vi "calcUkRef0.vi"(8 "error in (no error)":errorcluster, 9 "dofIdx":i32[](array[numeric]), 10 "Qx Array":dbl[][](array[numeric]), 11 "OptCtrl in":refnum<class "OptCtrl.lvclass">) -> (0 "error out":errorcluster, 2 "uk Array":dbl[](array[numeric]), 3 "OptCtrl out":refnum<class "OptCtrl.lvclass">)   [LabVIEW 2016, in "OptCtrl.lvclass"]
doc: "Calculate uk by referencing to \"0\". The offset will trace the real value and target for 0."
uses:
  OptCtrl.lvclass
  OptCtrl.lvclass/OptCtrl.ctl
  <vilib>/Analysis/baseanly.llb/Real A x B.vi
  <vilib>/Analysis/Matrix/Numeric/Conversions/Array To Matrix - RA2.vi
  Utility/getSubArray1D.vi
  <vilib>/Analysis/Matrix/Numeric/Add/Add - RM,RM.vi
  <vilib>/Analysis/Matrix/Numeric/Conversions/Matrix To Array - RM.vi
  <vilib>/Analysis/Matrix/NI_Matrix.lvlib
  <vilib>/Analysis/NI_AALBase.lvlib
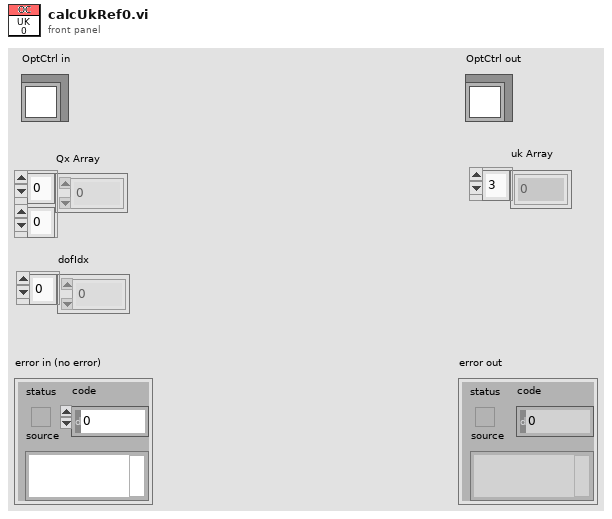
[diagram p1: front panel]
types:
  T1 = typedef "NI_Matrix.lvlib/RealMatrix.ctl" = dbl[][]
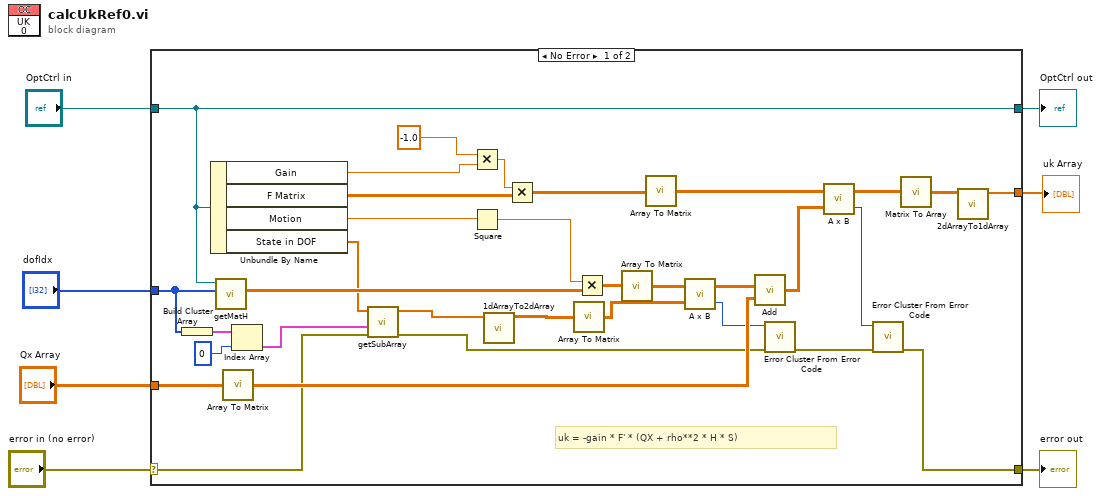
[diagram p0: block diagram]
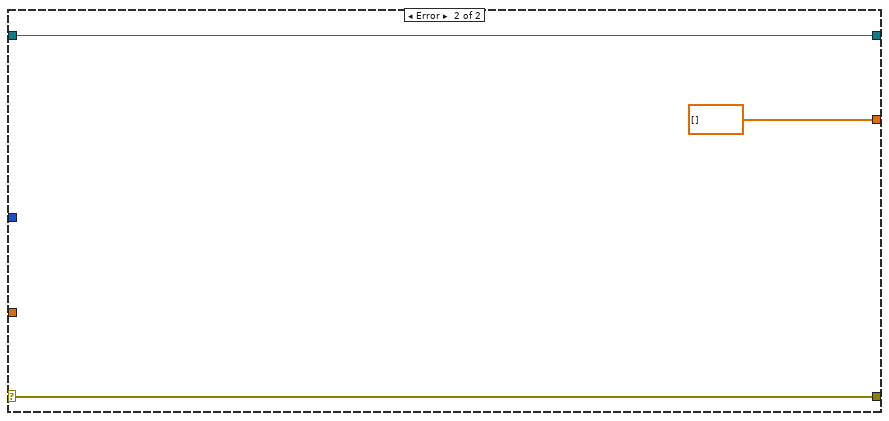
[diagram p2: hidden frame]
diagram:
  n1 = case shown="No Error" "error in (no error)" {
    selector: "error in (no error)" -> [w10 w43]
    tunnel: [w16 w43] -> w6
    tunnel: [w34 w42] -> w4
    tunnel: "OptCtrl in" -> [w34 w42]
    tunnel: "dofIdx" -> [w14 _]
    tunnel: "Qx Array" -> [w27 _]
    tunnel: [w20 dbl[] [] ("1D Array")] -> w1
    frame No Error {
      # "uk = -gain * F' * (QX + rho**2 * H * S)"
      n2 = Build Cluster Array(w14) -> (w13:cluster{"dofIdx":i32[]}[])
      n3 = Unbundle By Name(w34) -> ("Gain"=w39:dbl, "F Matrix"=w37:dbl[][], "Motion"=w35:dbl, "State in DOF"=w15:dbl[])
      n4 = call "getMatH.vi"("dofIdx"=w14, "OptCtrl in"=w34) -> ("Matrix H"=w32:dbl[][])  [unwired: 7 in, 2 out]
      n5 = call-poly <vilib>:"Array To Matrix.vi"("Real 2D Array"=w27) -> ("Real Matrix"=w25:T1)
      n6 = Index Array(array=w13, index=0) -> (element=w11:cluster{"dofIdx":i32[]})
      n7 = call-poly "getSubArray.vi"("error in (no error)"=w10, "Index Array Cluster"=w11, "1D Array"=w15) -> ("error out"=w9:errorcluster, "Sub-Array"=w8:dbl[])  [unwired: 7 in]
      n8 = Multiply(x=-1.0, y=w39) -> (x*y=w38:dbl)
      n9 = Square(x=w35) -> (x^2=w33:dbl)
      n10 = call "1dArrayTo2dArray.vi"("1D Array"=w8) -> ("2D Array"=w30:dbl[][])  [unwired: 10 in]
      n11 = Multiply(x=w38, y=w37) -> (x*y=w36:dbl[][])
      n12 = call-poly <vilib>:"Array To Matrix.vi"("Real 2D Array"=w30) -> ("Real Matrix"=w28:T1)
      n13 = Multiply(x=w33, y=w32) -> (x*y=w31:dbl[][])
      n14 = call-poly <vilib>:"Array To Matrix.vi"("Real 2D Array"=w31) -> ("Real Matrix"=w29:T1)
      n15 = call-poly <vilib>:"Array To Matrix.vi"("Real 2D Array"=w36) -> ("Real Matrix"=w24:T1)
      n16 = call-poly <vilib>:"A x B.vi"("B"=w28, "A"=w29) -> ("error"=w19:i32, "A x B"=w26:T1)
      n17 = call-poly <vilib>:"Add.vi"("Real Matrix B"=w25, "Real Matrix A"=w26) -> ("A + B"=w23:T1)
      n18 = call <vilib>:"Error Cluster From Error Code.vi"("error in (no error)"=w9, "error code (0)"=w19) -> ("error out"=w17:errorcluster)  [unwired: 7 in]
      n19 = call-poly <vilib>:"A x B.vi"("B"=w23, "A"=w24) -> ("error"=w18:i32, "A x B"=w22:T1)
      n20 = call <vilib>:"Error Cluster From Error Code.vi"("error in (no error)"=w17, "error code (0)"=w18) -> ("error out"=w16:errorcluster)  [unwired: 7 in]
      n21 = call-poly <vilib>:"Matrix To Array.vi"("Real Matrix"=w22) -> ("Real 2D Array"=w21:dbl[][])
      n22 = call "2dArrayTo1dArray.vi"("2D Array"=w21) -> ("1D Array"=w20:dbl[])  [unwired: 10 in]
    }
    frame Error {
    }
  }
  "error out" <- w6
  "OptCtrl out" <- w4
  "uk Array" <- w1
